vi "LC DB Close.vi"(8 "error in (no error)":errorcluster caption="错误输入（无错误）", 11 "DB Ref In":T1) -> (0 "error out":errorcluster caption="错误输出")   [LabVIEW 2020]
uses:
  <vilib>/addons/database/Connection.llb/Conn ObjectReference.ctl
  <vilib>/addons/database/NI_Database_API.lvlib
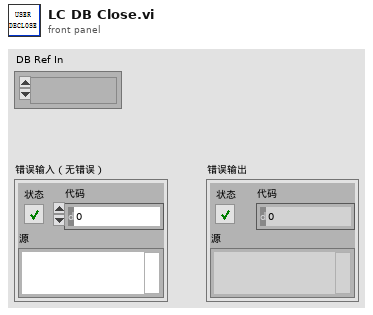
[diagram p1: front panel]
types:
  T1 = typedef "NI_Database_API.lvlib/Conn ObjectReference.ctl" = refnum<k1>
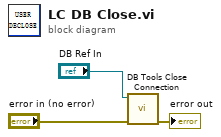
[diagram p0: block diagram]
diagram:
  n1 = call <vilib>:"DB Tools Close Connection.vi"("error in (no error)"="error in (no error)", "connection reference"="DB Ref In") -> ("error out"=→"error out":errorcluster)  [unwired: 5 in]
